vi "Event Text For Unregister One.vi"(6 "hotel":string, 9 "guest":string, 10 "zero registrations remaining?":bool, 11 "not registered?":bool) -> (3 "message":string)   [LabVIEW 2023]
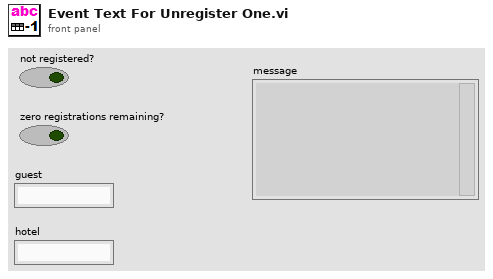
[diagram p1: front panel]
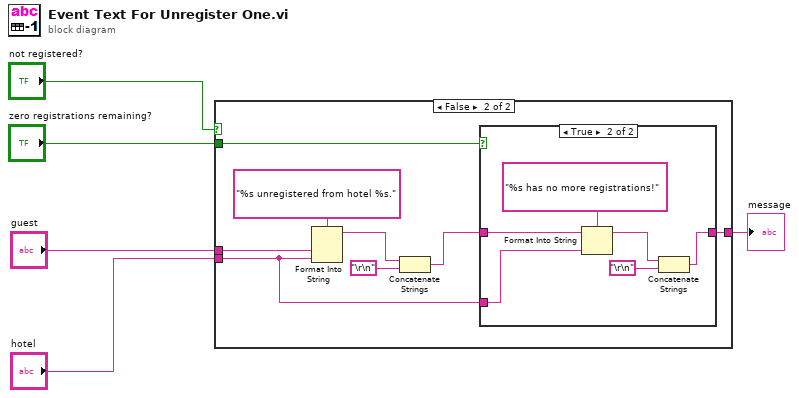
[diagram p0: block diagram]
diagram:
  n1 = case shown="False" "not registered?" {
    tunnel: "guest" -> [_ w12]
    tunnel: "hotel" -> [_ w9]
    tunnel: [_ w10] -> w3
    tunnel: "zero registrations remaining?" -> [_ w11]
    frame True {
      # "Not bothering to produce a message for every individual hotel. Caller will provide an aggregated message if the guest is not registered for any hotel."
    }
    frame False {
      n2 = Format Into String(format string="%s unregistered from hotel %s." ("L10n_message 1"), w12, w9) -> (resulting string=w7:string)  [unwired: 2 in, 1 out]
      n3 = Concatenate Strings(w7, "\r\n") -> (w6:string)
      n4 = case shown="True" w11 {
        tunnel: w6 -> [w14 w18]
        tunnel: [w14 w15] -> w10
        tunnel: w9 -> [_ w19]
        frame False {
        }
        frame True {
          n5 = Format Into String(format string="%s has no more registrations!" ("L10n_message 2"), initial string=w18, w19) -> (resulting string=w16:string)  [unwired: 1 in, 1 out]
          n6 = Concatenate Strings(w16, "\r\n") -> (w15:string)
        }
      }
    }
  }
  "message" <- w3
